vi "Gaussian_PeakFitter.vi"(9 "Y array in":dbl[](array[numeric]), 10 "Peak Threshold":dbl format="%p", 11 "X array in":dbl[](array[numeric])) -> (1 "Amplitudes":dbl[](array[numeric]), 2 "peak detection locations":dbl[](array[numeric]), 3 "FWHM":dbl[](array[numeric]))   [LabVIEW 2016]
uses:
  <vilib>/Analysis/1siggen.llb/Ramp Pattern by Samples.vi
  <vilib>/Analysis/2dsp.llb/1D Convolution (DBL).vi
  <vilib>/Analysis/NI_AAL_SigProc.lvlib
  <vilib>/Analysis/NI_AALBase.lvlib
  <vilib>/Analysis/6fits.llb/Curve Fitting Criteria.ctl
  <vilib>/Analysis/NI_AALPro.lvlib
panel:
  out "FWHM start value":dbl[](array[numeric])
  out "FWHM end y value":dbl[](array[numeric])
  out "half peak amps":dbl[](array[numeric])
  out "FWHM start":dbl[](array[numeric])
  out "FWHM end":dbl[](array[numeric])
  out "some of the half-peak X values":dbl[](array[numeric])
  out "error":i32
  out "size original":i32
  out "size(s)":i32
  in  "peak fitting width":i32=3 min=3
  out "peak detection errors":i32
  in  "balance parameter":dbl format="%#_20g"
  out "y size at the beginning":dbl
  out "spline error":i32
  in  "Smoothing Type":T1(ring)
  out "raw in":cluster{"Y array":dbl[], "X array":dbl[]}(graph)
  out "Raw + Gaussians":T2(graph)
  out "X step":dbl
  out "best gassian fits":T2(graph)
  out "Gaussian Info Array":T3(array[cluster])
  out "Peak Detection Voltage Values":dbl[](array[numeric])
  out "smoothed":cluster{"Y array":dbl[], "X array":dbl[]}(graph)
  out "Y (out)":dbl[](array[numeric])
  out "X ramped (out)":dbl[](array[numeric])
  out "x size at beginnning":dbl
  out "Y size":i32
  out "X size":i32
  out "end":dbl
  out "start":dbl
  out "offset":dbl
  # "0.999999899999989394"
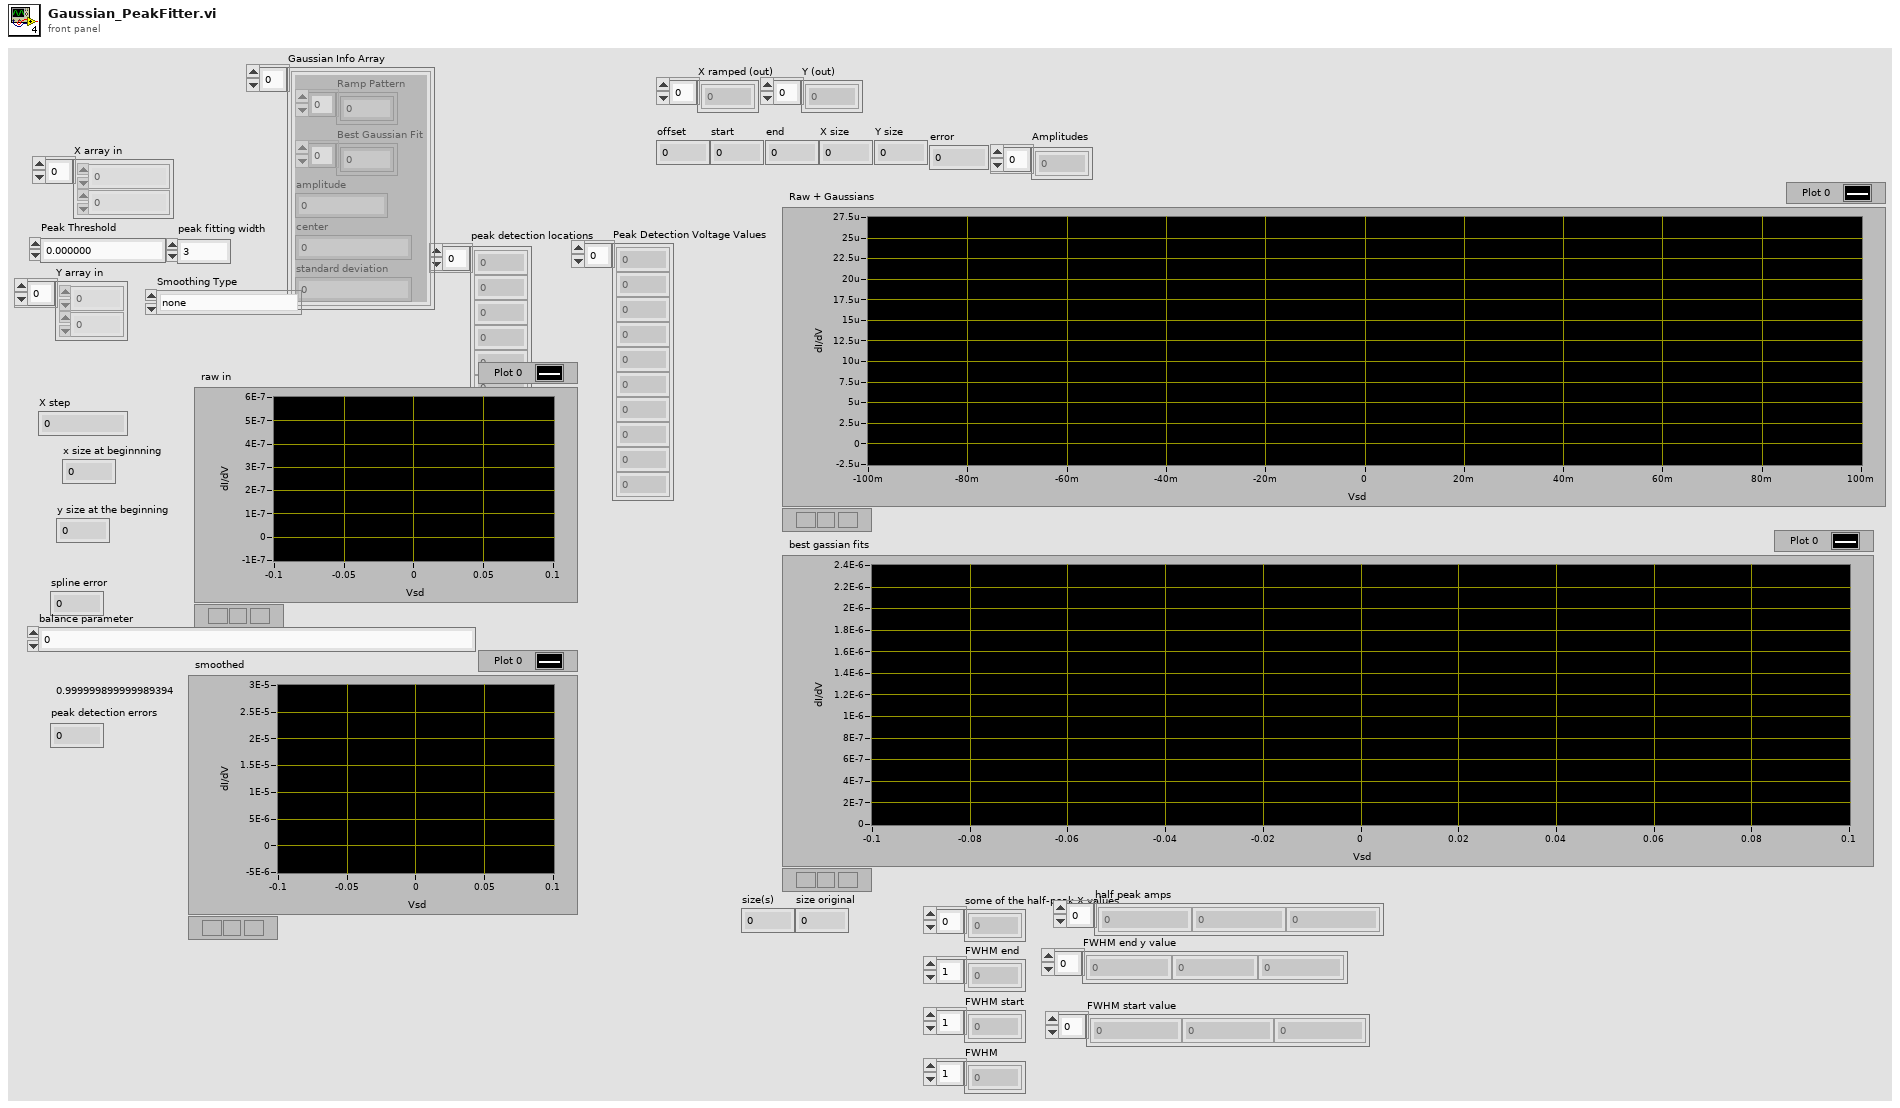
[diagram p1: front panel]
types:
  T1 = enum16{"none", "spline fit", "gaussian convolution"}
  T2 = cluster{"Ramp Pattern":dbl[], "Best Gaussian Fit":dbl[]}[]
  T3 = cluster{"Ramp Pattern":dbl[], "Best Gaussian Fit":dbl[], "amplitude":dbl, "center":dbl, "standard deviation":dbl}[]
  T4 = cluster{"amp min":dbl, "amp max":dbl, "center min":dbl, "center max":dbl, "deviation min":dbl, "deviation max":dbl, "offset min":dbl, "offset max":dbl}
  T5 = cluster{"initial amplitude":dbl, "initial center":dbl, "initial standard deviation":dbl, "offset":dbl}
  T6 = typedef "NI_AALPro.lvlib/Curve Fitting Criteria.ctl" = u16
  T7 = cluster{"Ramp Pattern":dbl[], "Best Gaussian Fit":dbl[], "amplitude":dbl, "center":dbl, "standard deviation":dbl}
  T8 = cluster{"Ramp Pattern":dbl[], "Best Gaussian Fit":dbl[]}
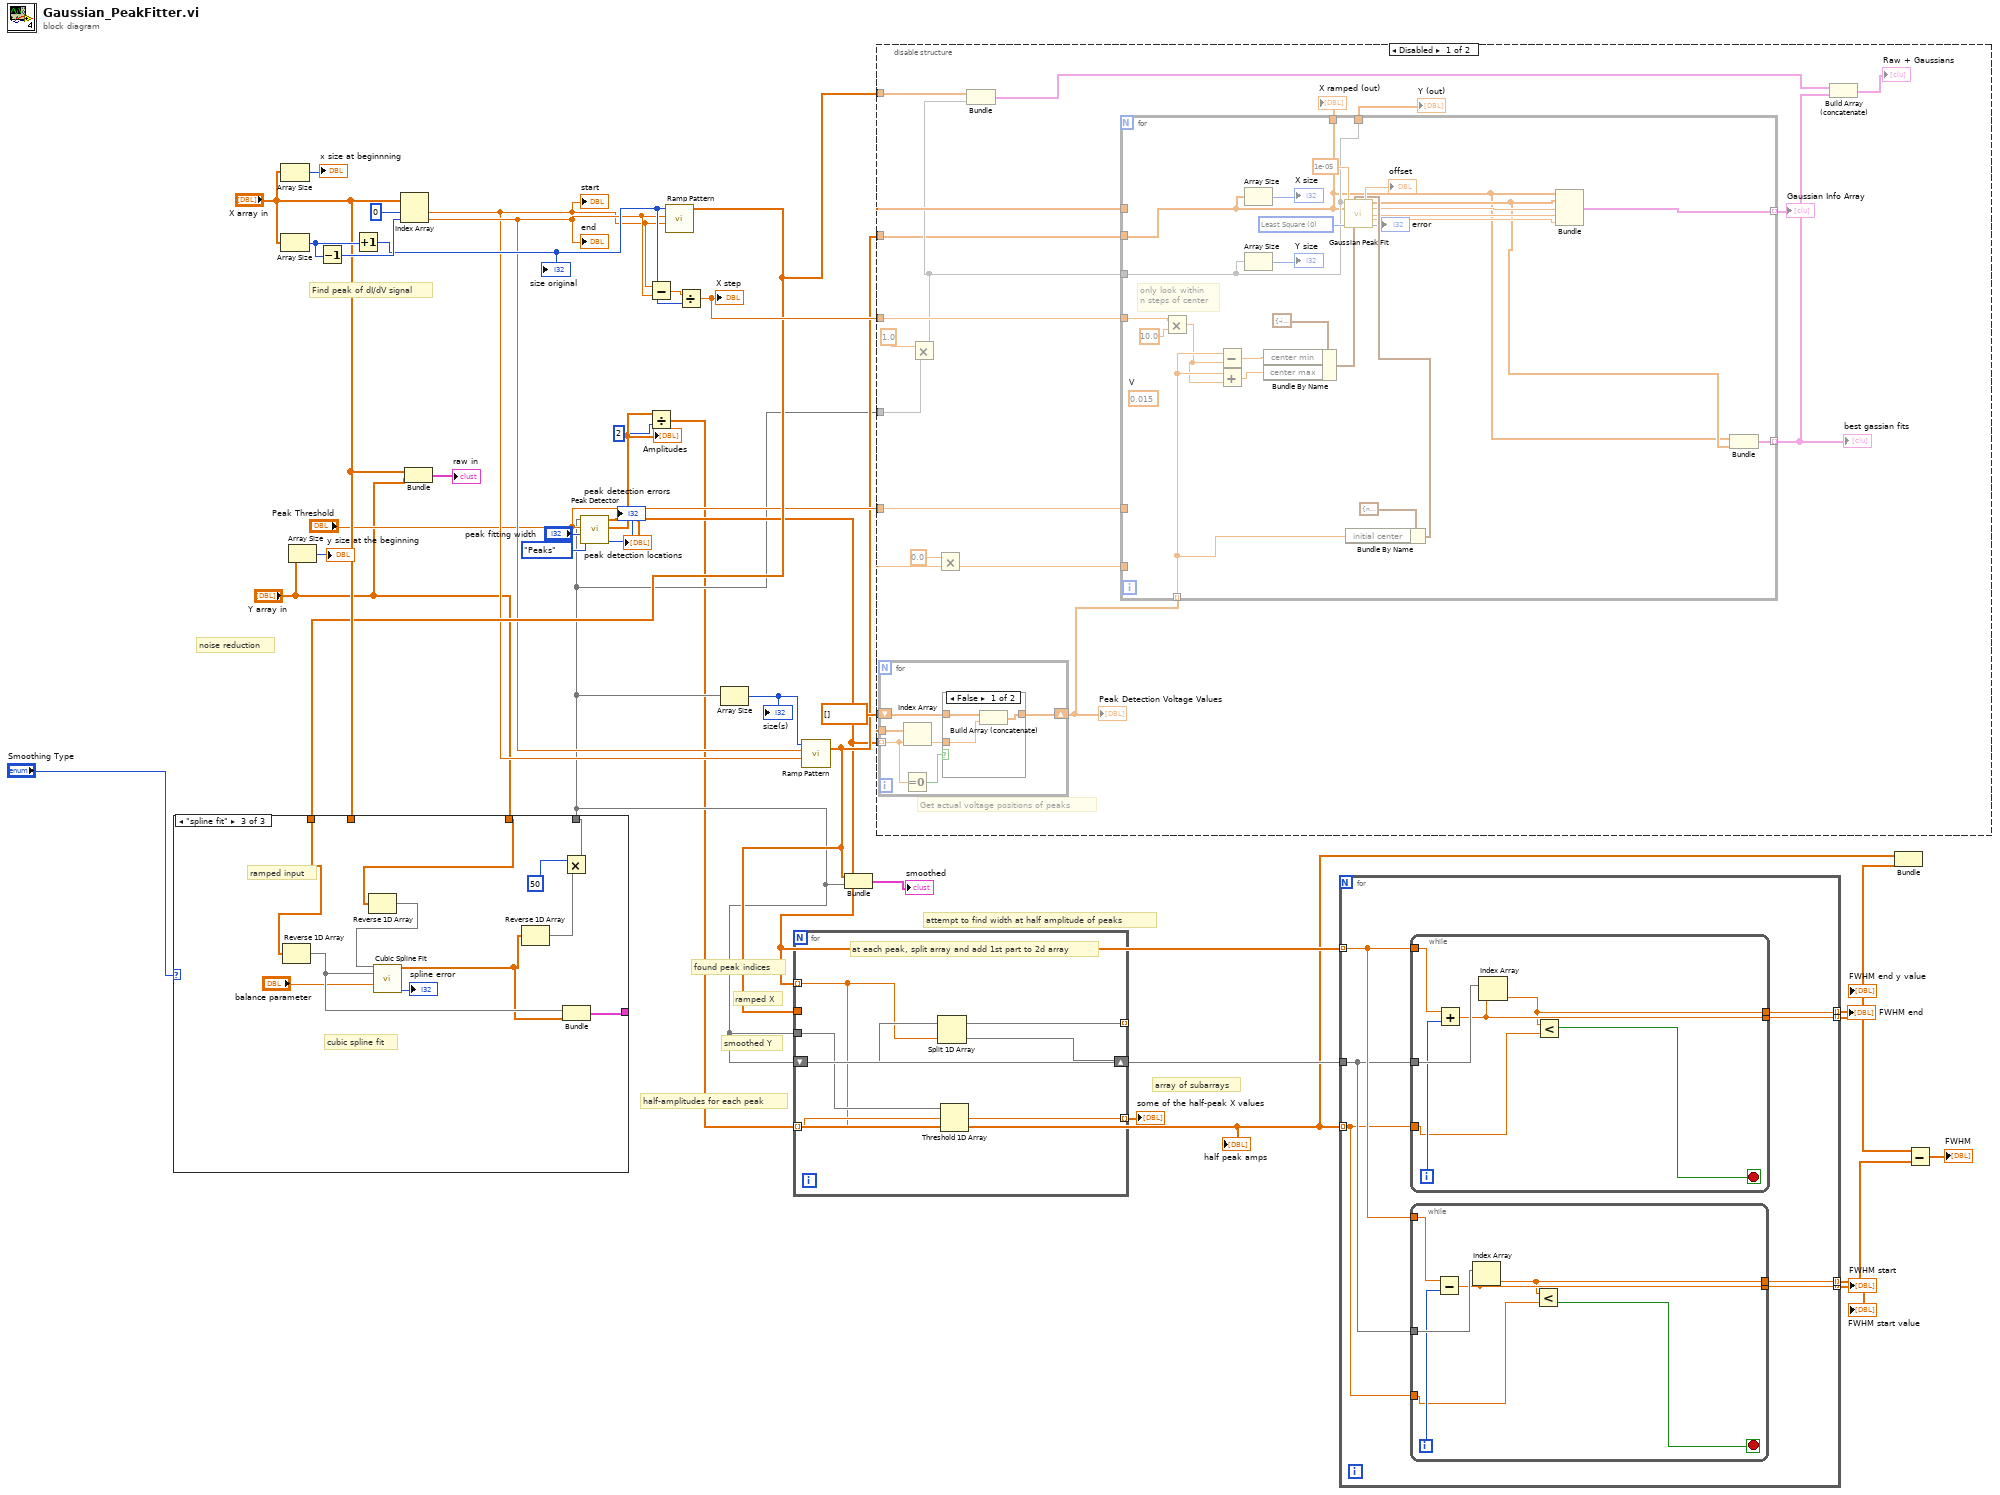
[diagram p0: block diagram]
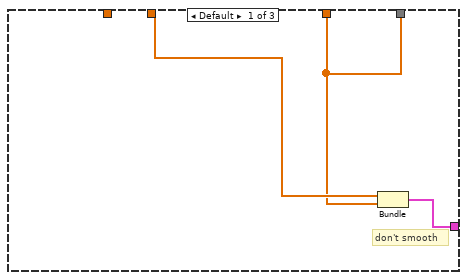
[diagram p4: hidden frame]
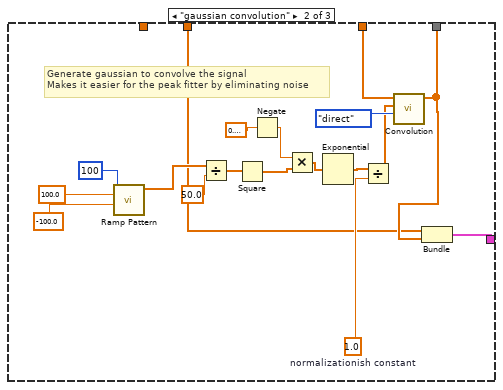
[diagram p5: hidden frame]
diagram:
  # "half-amplitudes for each peak"
  # "array of subarrays"
  # "found peak indices"
  # "ramped X"
  # "smoothed Y"
  # "attempt to find width at half amplitude of peaks"
  # "noise reduction"
  # "Find peak of dI/dV signal"
  n1 = Array Size(array="X array in") -> (size(s)=→"x size at beginnning":i32)
  n2 = Array Size(array="X array in") -> (size(s)=w33:i32)
  n3 = Array Size(array="Y array in") -> (size(s)=→"y size at the beginning":i32)
  n4 = Decrement(x=w33) -> (x-1=w32:i32)
  n5 = Increment(x=w33) -> (x+1=w29:i32)
  "size original" <- w29
  n6 = Index Array(array="X array in", index #1=0 ("index"), index #2=w32) -> (element #1=w17:dbl, element #2=w18:dbl)
  "start" <- w17
  "end" <- w18
  n7 = Bundle("X array in"="X array in", "Y array in"="Y array in") -> (→"raw in":cluster{"X array in":dbl[], "Y array in":dbl[]})  [unwired: 1 in]
  n8 = Subtract(x=w17, y=w18) -> (x-y=w28:dbl)
  n9 = call-poly <vilib>:"Ramp Pattern.vi"("start"=w17, "end"=w18, "samples"=w29) -> ("Ramp Pattern"=w22:dbl[])  [unwired: 7 in, 1 out]
  n10 = case shown="\"spline fit\"" "Smoothing Type" {
    tunnel: [w36 w45 w57] -> w5
    tunnel: [w35 w43 w66] -> _
    tunnel: "X array in" -> [w37 w39 _]
    tunnel: "Y array in" -> [w36 w38 w64]
    tunnel: w22 -> [_ _ w62]
    frame Default {
      # "don't smooth"
      n11 = Bundle("X array in"=w37, "Y array in"=w36) -> (w35:cluster{"X array in":dbl[], "Y array in":dbl[]})  [unwired: 1 in]
    }
    frame "gaussian convolution" {
      w40 = 1.0  # normalizationish constant
      # "Generate gaussian to convolve the signal\nMakes it easier for the peak fitter by eliminating noise"
      n12 = call-poly <vilib>:"Ramp Pattern.vi"("start"=-100.0, "end"=100.0, "samples"=100) -> ("Ramp Pattern"=w52:dbl[])  [unwired: 7 in, 1 out]
      n13 = Divide(x=w52, y=50.0 ("end")) -> (x/y=w50:dbl[])
      n14 = Square(x=w50) -> (x^2=w49:dbl[])
      n15 = Negate(x=0.6931471805599453) -> (-x=w48:dbl)
      n16 = Multiply(x=w48, y=w49) -> (x*y=w46:dbl[])
      n17 = Exponential(1:w46) -> (0:w41:dbl[])
      n18 = Divide(x=w41, y=w40) -> (x/y=w42:dbl[])
      n19 = call-poly <vilib>:"Convolution.vi"("algorithm"=enum32{"direct", "frequency domain"}."direct", "Y"=w42, "X"=w38) -> ("X * Y"=w45:dbl[])  [unwired: 7 in, 1 out]
      n20 = Bundle("X array in"=w39, "X * Y"=w45) -> (w43:cluster{"X array in":dbl[], "X * Y":dbl[]})  [unwired: 1 in]
    }
    frame "spline fit" {
      # "ramped input"
      # "cubic spline fit"
      n21 = Reverse 1D Array(array=w62) -> (reversed array=w61:dbl[])
      n22 = Reverse 1D Array(array=w64) -> (reversed array=w63:dbl[])
      n23 = call <vilib>:"Cubic Spline Fit.vi"("Y"=w63, "X"=w61, "balance parameter"="balance parameter") -> ("Best Cubic Spline Fit"=w58:dbl[], "error"=→"spline error":i32)  [unwired: 11 in]
      n24 = Reverse 1D Array(array=w58) -> (reversed array=w59:dbl[])
      n25 = Multiply(x=50, y=w59) -> (x*y=w57:dbl[])
      n26 = Bundle(w61, "Best Cubic Spline Fit"=w58) -> (w66:cluster{dbl[], "Best Cubic Spline Fit":dbl[]})  [unwired: 1 in]
    }
  }
  n27 = call <vilib>:"Peak Detector.vi"("peaks/valleys"=enum32{"Peaks", "Valleys"}."Peaks", "width"="peak fitting width", "threshold"="Peak Threshold", "X"=w5) -> ("error"=→"peak detection errors":i32, "Amplitudes"=w12:dbl[], "Locations"=w8:dbl[])  [unwired: 3 in, 2 out]
  "peak detection locations" <- w8
  "Amplitudes" <- w12
  n28 = Divide(x=w12, y=2) -> (x/y=w4:dbl[])
  "half peak amps" <- w4
  n29 = Divide(x=w28, y=w29) -> (x/y=w27:dbl)
  "X step" <- w27
  n30 = Array Size(array=w5) -> (size(s)=w16:i32)
  "size(s)" <- w16
  n31 = call-poly <vilib>:"Ramp Pattern.vi"("start"=w17, "end"=w18, "samples"=w16) -> ("Ramp Pattern"=w10:dbl[])  [unwired: 7 in, 1 out]
  n32 = for {
    tunnel: w5 -> [w70]
    tunnel: w10 -> [_]
    tunnel: w8 -> [w68] mode=indexing
    shift-right: [w72] -> _
    shift-left: w5 -> [w71]
    tunnel: [w73] -> _ mode=indexing
    tunnel: w4 -> [w69] mode=indexing
    tunnel: [w67] -> w9 mode=indexing
    # "at each peak, split array and add 1st part to 2d array"
    n33 = Split 1D Array(array=w71, index=w68) -> (first subarray=w73:dbl[], second subarray=w72:dbl[])
    n34 = Threshold 1D Array(1:w68, 2:w69, 3:w70) -> (0:w67:dbl)
  }
  "some of the half-peak X values" <- w9
  n35 = Bundle("Ramp Pattern"=w10, "X * Y"=w5) -> (→"smoothed":cluster{"Ramp Pattern":dbl[], "X * Y":dbl[]})  [unwired: 1 in]
  n36 = disable-structure shown="Disabled" {
    disable-tunnel: dbl[] [] -> [w89 _]
    disable-tunnel: w27 -> [w86 _]
    disable-tunnel: w22 -> [w82 _]
    disable-tunnel: "Peak Threshold" -> [w79 _]
    disable-tunnel: w10 -> [w76 _]
    disable-tunnel: w8 -> [w75 _]
    disable-tunnel: w5 -> [w74 _]
    frame Disabled {
      # "Get actual voltage positions of peaks"
      n37 = for {
        tunnel: w75 -> [w94] mode=indexing
        shift-right: [w92] -> w88
        shift-left: w89 -> [w97]
        tunnel: w76 -> [w96]
        n38 = Equal To 0?(x=w94) -> (x = 0?=w93:bool)
        n39 = Index Array(array=w96, index=w94) -> (element=w95:dbl)
        n40 = case shown="False" w93 {
          tunnel: [w100 w101] -> w92
          tunnel: w97 -> [w99 w101]
          tunnel: w95 -> [w98 _]
          frame False {
            n41 = Build Array (concatenate)(w99, w98) -> (w100:dbl[])
          }
          frame True {
          }
        }
      }
      "Peak Detection Voltage Values" <- w88
      n42 = Multiply(x=1.0, y=w74) -> (x*y=w81:dbl[])
      n43 = Multiply(x=0.0, y=w79) -> (x*y=w78:dbl)
      n44 = Bundle("Ramp Pattern"=w82, w81) -> (w85:cluster{"Ramp Pattern":dbl[], dbl[]})  [unwired: 1 in]
      n45 = for {
        tunnel: w81 -> [w105]
        tunnel: w82 -> [_]
        tunnel: w79 -> [_]
        tunnel: [w102] -> w91
        tunnel: [w105] -> w90
        tunnel: w88 -> [w108] mode=indexing
        tunnel: [w116] -> w87 mode=indexing
        tunnel: [w115] -> w83 mode=indexing
        tunnel: w86 -> [w111]
        tunnel: w78 -> [_]
        tunnel: w76 -> [w102]
        (unwired) 0.015  # V
        w124 = T6 0 items=["Least Square", "Least Absolute Residual", "Bisquare"] ("method")
        # "only look within\nn steps of center"
        n46 = Multiply(x=w111, y=10.0) -> (x*y=w107:dbl)
        n47 = Subtract(x=w108, y=w107) -> (x-y=w110:dbl)
        n48 = Add(x=w108, y=w107) -> (x+y=w109:dbl)
        n49 = Array Size(array=w102) -> (size(s)=→"X size":i32)
        n50 = Array Size(array=w105) -> (size(s)=→"Y size":i32)
        n51 = Bundle By Name(cluster=T4 {"amp min"=-inf, "amp max"=inf, "center min"=-inf, "center max"=inf, "deviation min"=-inf, "deviation max"=inf, "offset min"=0.0, "offset max"=0.0} ("parameter bounds"), "center min"=w110, "center max"=w109) -> (w104:T4)
        n52 = Bundle By Name(cluster=T5 {"initial amplitude"=nan, "initial center"=nan, "initial standard deviation"=nan, "offset"=nan} ("initial guess"), "initial center"=w108) -> (w120:T5)
        n53 = call <vilib>:"Gaussian Peak Fit.vi"("Y"=w105, "initial guess"=w120, "X"=w102, "tolerance"=1e-05, "method"=w124, "parameter bounds"=w104) -> ("offset"=→"offset":dbl, "Best Gaussian Fit"=w114:dbl[], "amplitude"=w119:dbl, "center"=w118:dbl, "standard deviation"=w117:dbl, "error"=→"error":i32)  [unwired: 3 in, 1 out]
        n54 = Bundle("Ramp Pattern"=w102, "Best Gaussian Fit"=w114, "amplitude"=w119, "center"=w118, "standard deviation"=w117) -> (w116:T7)  [unwired: 1 in]
        n55 = Bundle("Ramp Pattern"=w102, "Best Gaussian Fit"=w114) -> (w115:T8)  [unwired: 1 in]
      }
      "X ramped (out)" <- w91
      "Y (out)" <- w90
      "Gaussian Info Array" <- w87
      "best gassian fits" <- w83
      n56 = Build Array (concatenate)(w85, w83) -> (→"Raw + Gaussians":T2)
    }
    frame Enabled {
    }
  }
  n57 = for {
    tunnel: w5 -> [w130]
    tunnel: w4 -> [w129] mode=indexing
    tunnel: w8 -> [w131] mode=indexing
    tunnel: [w132] -> w3 mode=indexing
    tunnel: [w128] -> w7 mode=indexing
    tunnel: [w127] -> w2 mode=indexing
    tunnel: [w126] -> w1 mode=indexing
    n58 = while {
      tunnel: w130 -> [w139]
      tunnel: w129 -> [w136]
      tunnel: w131 -> [w138]
      tunnel: [w134] -> w128
      tunnel: [w133] -> w126
      i -> [w137]
      stop <- w135 stop-if-true
      n59 = Subtract(x=w138, y=w137) -> (x-y=w134:dbl)
      n60 = Index Array(array=w139, index=w134) -> (element=w133:dbl)
      n61 = Less?(x=w133, y=w136) -> (x < y?=w135:bool)
    }
    n62 = while {
      tunnel: w130 -> [w146]
      tunnel: w129 -> [w143]
      tunnel: w131 -> [w145]
      tunnel: [w141] -> w132
      tunnel: [w140] -> w127
      i -> [w144]
      stop <- w142 stop-if-true
      n63 = Add(x=w145, y=w144) -> (x+y=w141:dbl)
      n64 = Index Array(array=w146, index=w141) -> (element=w140:dbl)
      n65 = Less?(x=w140, y=w143) -> (x < y?=w142:bool)
    }
  }
  "FWHM end" <- w3
  "FWHM start" <- w7
  "FWHM end y value" <- w2
  "FWHM start value" <- w1
  n66 = Bundle(w4, w3) -> ()  [unwired: 1 in, 1 out]
  n67 = Subtract(x=w3, y=w7) -> (x-y=→"FWHM":dbl[])
